vi "I-SRC Configure (26XX).vi"(5 "Voltage Limit":dbl, 7 "Current Level":dbl, 8 "error in (no error)":errorcluster, 11 "VISA resource name in":refnum<visa-resource-name>) -> (0 "error out":errorcluster, 3 "VISA resource name out":refnum<visa-resource-name>)   [LabVIEW 2016, in "Hall Effect Library.lvlib"]
uses:
  Hall Effect Library.lvlib
  <instrlib>/KE26XX/KE26XX.lvlib
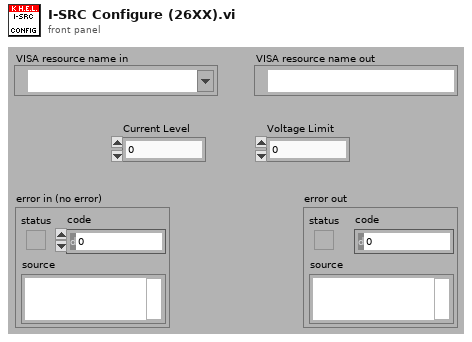
[diagram p1: front panel]
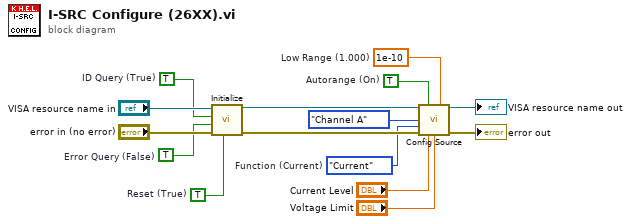
[diagram p0: block diagram]
diagram:
  w6 = 1e-10  # Low Range (1.000)
  w7 = TRUE  # Autorange (On)
  w8 = enum32{"Current", "Voltage"}."Current"  # Function (Current)
  w9 = TRUE  # Reset (True)
  w10 = TRUE  # Error Query (False)
  w11 = TRUE  # ID Query (True)
  n1 = call <instrlib>:"Initialize.vi"("Reset (True)"=w9, "error in (no error)"="error in (no error)", "Error Query (False)"=w10, "ID Query (True)"=w11, "VISA resource name"="VISA resource name in") -> ("error out"=w14:errorcluster, "VISA resource name out"=w15:refnum<visa-resource-name>)  [unwired: 1 in, 4 out]
  n2 = call <instrlib>:"Config Source.vi"("VISA resource name"=w15, "Autorange (On)"=w7, "Low Range (1.000)"=w6, "Channel (Channel A)"=enum32{"Channel A", "Channel B"}."Channel A", "Function (Current)"=w8, "error in"=w14, "Level (0.000)"="Current Level", "Limit (0.1)"="Voltage Limit") -> ("VISA resource name out"=→"VISA resource name out":refnum<visa-resource-name>, "error out"=→"error out":errorcluster)  [unwired: 3 in, 3 out]
